vi "SLSC_Example_AsyscRTEnginer.vi"(10 "Parameters":variant, 11 "Process":refnum<class "Process.lvclass">) -> ()   [LabVIEW 2015, in "SLSC Module Template Engine.lvlib"]
uses:
  SLSC Module Template Engine.lvlib
  <vilib>/NI/NIVS Inline Async API/_VS Inline Async API/Process/Process.lvclass
  Shared/Compiled.Settings
  Shared/SLSC Dynamic Channel.ctl
  Types/Async Engine State Control.ctl
  <vilib>/NI/NIVS Inline Async API/_VS Inline Async API/Process/Process.lvclass/Process.ctl
  <vilib>/NI/NIVS Inline Async API/_Data Access Engine/Access Type Classes/Read/Read.lvclass/Read.ctl
  <vilib>/NI/NIVS Inline Async API/_Data Access Engine/Access Type Classes/ReadWrite/ReadWrite.lvclass/ReadWrite.ctl
  <vilib>/NI/NIVS Inline Async API/_Data Access Engine/Access Type Classes/Write/Write.lvclass/Write.ctl
  <vilib>/NI/NIVS Inline Async API/_Data Access Engine/Data Access Engine/Methods/Read.Data.vi
  <vilib>/NI/NIVS Inline Async API/_Data Access Engine/Data Access Engine/Methods/Write.Data.vi
  <vilib>/NI/NIVS Inline Async API/_Data Access Engine/Data Access Engine/Methods/ReadWrite.Data.vi
  <vilib>/NI/NIVS Inline Async API/_VS Inline Async API/Process/Data Member Access/Read Data Access.vi
  <vilib>/NI/NIVS Inline Async API/_VS Inline Async API/Error Handling Process/SubVIs/Error.ConvertArray.vi
  <vilib>/NI/NIVS Inline Async API/_Data Access Engine/Access Type Classes/Read/Read.ProcessData.vi
  <vilib>/NI/NIVS Inline Async API/_Data Access Engine/Access Type Classes/Write/Write.ProcessData.vi
  SLSC_Determine_Resource.vi
  <vilib>/NI/NIVS Inline Async API/_Data Access Engine/Access Type Classes/ReadWrite/ReadWrite.ProcessData.vi
  <vilib>/SLSC/Commit Properties.vi
  <vilib>/SLSC/Commit Properties for Devices.vi
  <vilib>/SLSC/Set Generic Property.vi
  <vilib>/SLSC/Set Generic Property (U64).vi
  <vilib>/SLSC/Set Generic Property (U32).vi
  <vilib>/SLSC/Set Generic Property (String).vi
  <vilib>/SLSC/Set Generic Property (I64).vi
  <vilib>/SLSC/Set Generic Property (I32).vi
  <vilib>/SLSC/Set Generic Property (DBL).vi
  <vilib>/SLSC/Set Generic Property (Bool).vi
  <vilib>/SLSC/Close Session.vi
  <vilib>/SLSC/Get Generic Property.vi
  <vilib>/SLSC/Get Generic Property (U64).vi
  <vilib>/SLSC/Get Generic Property (U32).vi
  <vilib>/SLSC/Get Generic Property (String).vi
  <vilib>/SLSC/Get Generic Property (I64).vi
  <vilib>/SLSC/Get Generic Property (I32).vi
  <vilib>/SLSC/Get Generic Property (DBL).vi
  <vilib>/SLSC/Get Generic Property (Bool).vi
  <vilib>/SLSC/Execute Command.vi
  <vilib>/SLSC/Execute Phys Chan Command.vi
  <vilib>/SLSC/Execute Device Command.vi
  <vilib>/NI/NIVS Inline Async API/_Data Access Engine/Data Access Engine/Methods/ReadWrite.Lookup.vi
  <vilib>/NI/NIVS Inline Async API/_Data Access Engine/Data Access Engine/Methods/Read.Lookup.vi
  <vilib>/NI/NIVS Inline Async API/_Data Access Engine/Data Access Engine/Methods/Write.Lookup.vi
  Shared/Constants.vi
  <vilib>/NI/NIVS Inline Async API/_Data Access Engine/Data Access Engine/Data Access Engine.lvclass
  <vilib>/NI Veristand/Custom Device Tools/Custom Device Utility Library/Custom Device Utility Library.lvlib
  <vilib>/SLSC/SLSC.lvlib
  Shared/SLSC Module Template Shared.lvlib
  System Explorer/SLSC Module Template System Explorer.lvlib
panel:
  in  "LoopRate(ms)":u32=50
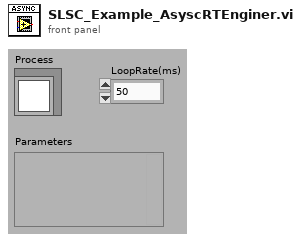
[diagram p1: front panel]
types:
  T1 = typedef "SLSC Module Template Engine.lvlib/Async Engine State Control.ctl" = enum16{"Initialize", "Configure", "Run", "Reset", "Shutdown"}
  T2 = typedef "SLSC Module Template Shared.lvlib/Compiled.Settings" = cluster{"Name":string, "SLSC IP Address":string, "Slot #":i32, "Configuration Data":cluster{"Properties":cluster{"Boolean Properties":cluster{"property":refnum<k21>, "Value":bool, "SLSC Item":refnum<k21>}[], "Double Properties":cluster{"property":refnum<k21>, "Double Write":dbl, "SLSC Item":refnum<k21>}[], "I32 Properties":cluster{"property":refnum<k21>, "Int32 Write":i32, "SLSC Item":refnum<k21>}[], "I64 Properties":cluster{"property":refnum<k21>, "Int64 Write":i64, "SLSC Item":refnum<k21>}[], "String Properties":cluster{"property":refnum<k21>, "String Write":string, "SLSC Item":refnum<k21>}[], "U32 Properties":cluster{"property":refnum<k21>, "UInt32 Write":u32, "SLSC Item":refnum<k21>}[], "U64 Properties":cluster{"property":refnum<k21>, "UInt64 Write":u64, "SLSC Item":refnum<k21>}[]}}, "SLSC Dynamic Inputs":T3[], "SLSC Dynamic Outputs":T3[], "SLSC Dynamic Commands":T3[]}
  T3 = typedef "SLSC Module Template System Explorer.lvlib/SLSC Dynamic Channel.ctl" = cluster{"SLSC Item":string, "property":string, "Data Type":enum16{"Bool", "Double", "I32", "I64", "String", "U32", "U64"}}
  T4 = typedef "Data Access Engine.lvlib/Data Access Engine.lvclass/Write.DVR.ctl" = refnum<data-value>
  T5 = typedef "Data Access Engine.lvlib/Data Access Engine.lvclass/Read.DVR.ctl" = refnum<data-value>
  T6 = typedef "Data Access Engine.lvlib/Data Access Engine.lvclass/ReadWrite.DVR.ctl" = refnum<data-value>
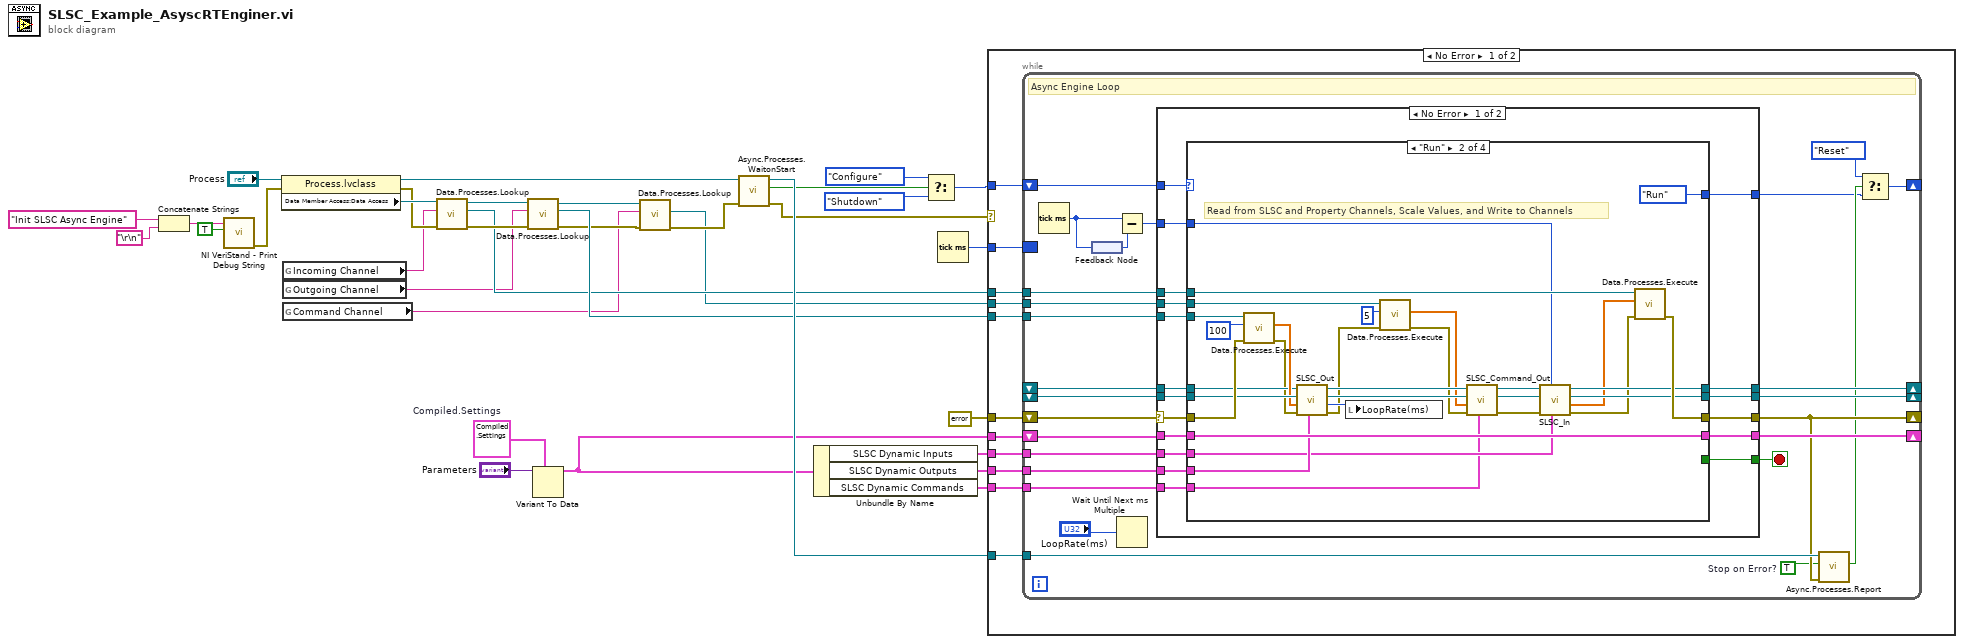
[diagram p0: block diagram]
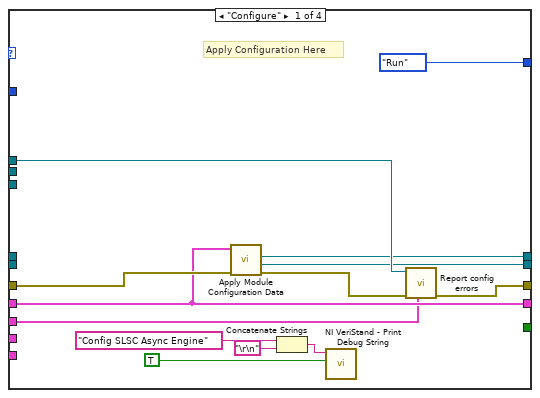
[diagram p2: hidden frame]
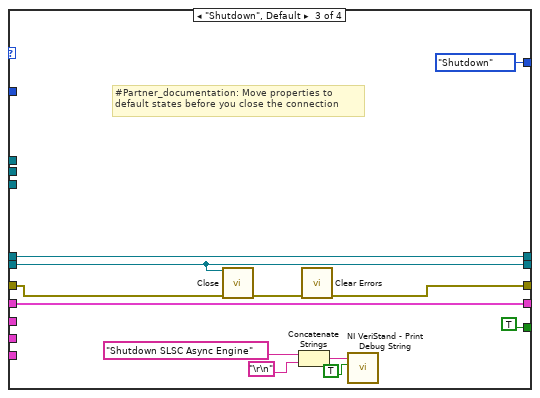
[diagram p3: hidden frame]
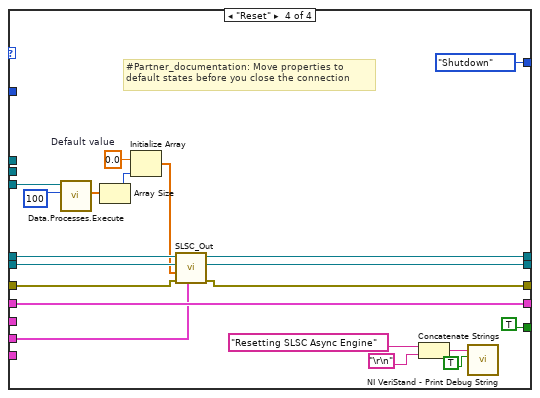
[diagram p4: hidden frame]
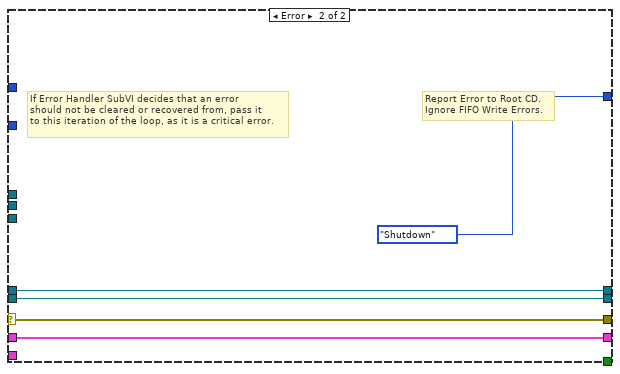
[diagram p5: hidden frame]
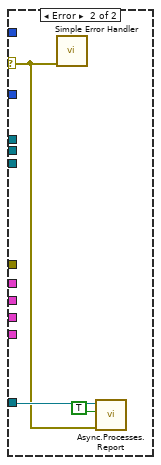
[diagram p6: hidden frame]
diagram:
  w23 = T2 {"Name"="", "SLSC IP Address"="", "Slot #"=0, "Configuration Data"={"Properties"={"Boolean Properties"=[], "Double Properties"=[], "I32 Properties"=[], "I64 Properties"=[], "String Properties"=[], "U32 Properties"=[], "U64 Properties"=[]}}, "SLSC Dynamic Inputs"=[], "SLSC Dynamic Outputs"=[], "SLSC Dynamic Commands"=[]}  # Compiled.Settings
  n1 = Concatenate Strings("Init SLSC Async Engine" ("Message"), "\r\n") -> (w20:string)
  n2 = call <vilib>:"NI VeriStand - Print Debug String.vi"("Add to log file? (T)"=TRUE, "Message"=w20) -> ("error out"=w7:errorcluster)  [unwired: 9 in]
  n3 = property class="Process.lvclass"(reference="Process", error in=w7) -> (reference out=w27:refnum<class "Process.lvclass">, error out=w25:errorcluster, "Data Member Access:Data Access"=w26:refnum<class "Data Access Engine.lvclass">)
  n4 = global read "Constants.vi" "Incoming Channel"() -> (w10:string)
  n5 = global read "Constants.vi" "Outgoing Channel"() -> (w9:string)
  n6 = global read "Constants.vi" "Command Channel"() -> (w2:string)
  n7 = call-poly <vilib>:"Data.Processes.Lookup.vi"("error in (no error)"=w25, "Name"=w10, "Data Access API in"=w26) -> ("error out"=w31:errorcluster, "Ref"=w30:T4, "Data Access API out"=w29:refnum<class "Data Access Engine.lvclass">)  [unwired: 5 in, 1 out]
  n8 = call-poly <vilib>:"Data.Processes.Lookup.vi"("error in (no error)"=w31, "Name"=w9, "Data Access API in"=w29) -> ("error out"=w4:errorcluster, "Ref"=w32:T5, "Data Access API out"=w5:refnum<class "Data Access Engine.lvclass">)  [unwired: 5 in, 1 out]
  n9 = Variant To Data(type=w23, Variant="Parameters") -> (data=w13:T2)  [unwired: 1 in, 1 out]
  n10 = call-poly <vilib>:"Data.Processes.Lookup.vi"("error in (no error)"=w4, "Name"=w2, "Data Access API in"=w5) -> ("error out"=w3:errorcluster, "Ref"=w1:T6)  [unwired: 5 in, 2 out]
  n11 = call <vilib>:"Async.Processes.WaitonStart.vi"("error in (no error)"=w3, "Process"=w27) -> ("error out"=w33:errorcluster, "Execute"=w17:bool, "Process out"=w34:refnum<class "Process.lvclass">)  [unwired: 7 in]
  n12 = Unbundle By Name(w13) -> ("SLSC Dynamic Inputs"=w12:T3[], "SLSC Dynamic Outputs"=w11:T3[], "SLSC Dynamic Commands"=w6:T3[])
  n13 = Select(t=Async_Engine_State_Control."Configure", s=w17, f=Async_Engine_State_Control."Shutdown") -> (s? t:f=w14:T1)
  n14 = Tick Count (ms)() -> (millisecond timer value=w8:u32)
  n15 = case shown="No Error" w33 {
    selector: w33 -> [_ w171]
    tunnel: w34 -> [w45 w172]
    tunnel: w30 -> [w44 _]
    tunnel: w32 -> [w43 _]
    tunnel: w13 -> [w37 _]
    tunnel: errorcluster {"status"=FALSE, "code"=0, "source"=""} ("error IO") -> [w42 _]
    tunnel: w14 -> [w41 _]
    tunnel: w12 -> [w40 _]
    tunnel: w11 -> [w39 _]
    tunnel: w8 -> [w38 _]
    tunnel: w6 -> [w36 _]
    tunnel: w1 -> [w35 _]
    frame No Error {
      n16 = while {
        shift-right: [w61] -> _
        shift-left: w42 -> [w70]
        shift-right: [w49] -> _
        shift-left: w41 -> [w69]
        shift-right: [w68] -> _
        shift-left: w37 -> [w67]
        shift-right: [w66] -> _
        shift-left: _ -> [w65]
        tunnel: w43 -> [w64]
        tunnel: w44 -> [w63]
        tunnel: w45 -> [w62]
        tunnel: w40 -> [w60]
        tunnel: w39 -> [w59]
        shift-right: [w58] -> _
        shift-left: _ -> [w57]
        border: w38 -> [_]
        tunnel: w36 -> [w47]
        tunnel: w35 -> [w46]
        stop <- w52 stop-if-true
        w56 = TRUE  # Stop on Error?
        # "Async Engine Loop"
        n17 = Tick Count (ms)() -> (millisecond timer value=w55:u32)
        n18 = feedback-in #1(w55) -> ()
        n19 = feedback #1() -> (w54:u32)
        n20 = Subtract(x=w55, y=w54) -> (x-y=w53:u32)
        n21 = Wait Until Next ms Multiple(millisecond multiple="LoopRate(ms)") -> ()  [unwired: 1 out]
        n22 = case shown="No Error" w70 {
          selector: w70 -> [w88 w166]
          tunnel: [w81 w166] -> w61
          tunnel: w69 -> [w89 _]
          tunnel: [w82 Async_Engine_State_Control."Shutdown"] -> w50
          tunnel: [w87 _] -> w52
          tunnel: [w86 w169] -> w68
          tunnel: w67 -> [w85 w169]
          tunnel: [w84 w168] -> w66
          tunnel: w65 -> [w83 w168]
          tunnel: w64 -> [w80 _]
          tunnel: w63 -> [w79 _]
          tunnel: w60 -> [w78 _]
          tunnel: w59 -> [w77 _]
          tunnel: [w76 w165] -> w58
          tunnel: w57 -> [w75 w165]
          tunnel: w53 -> [w74 _]
          tunnel: w47 -> [w73 _]
          tunnel: w46 -> [w72 _]
          frame No Error {
            n23 = case shown="\"Run\"" w89 {
              tunnel: w88 -> [w102 w129 w133 w145]
              tunnel: [w93 w128 w136 w157] -> w81
              tunnel: [Async_Engine_State_Control."Run" Async_Engine_State_Control."Run" Async_Engine_State_Control."Shutdown" Async_Engine_State_Control."Shutdown"] -> w82
              tunnel: [_ _ TRUE TRUE] -> w87
              tunnel: [w96 w132 w143 w163] -> w86
              tunnel: w85 -> [w96 w132 w143 w163]
              tunnel: [w90 w120 w134 w150] -> w84
              tunnel: w83 -> [_ w125 w134 w151]
              tunnel: w80 -> [_ w130 _ w155]
              tunnel: w79 -> [w94 w126 _ _]
              tunnel: w78 -> [w92 w118 _ _]
              tunnel: w77 -> [_ w123 _ w154]
              tunnel: [w91 w121 w135 w152] -> w76
              tunnel: w75 -> [_ w122 w135 w153]
              tunnel: w74 -> [_ w116 _ _]
              tunnel: w73 -> [_ w106 _ _]
              tunnel: w72 -> [_ w114 _ _]
              frame "Configure" {
                # "Apply Configuration Here"
                n24 = call "Apply Module Configuration Data.vi"("Error In"=w102, "Compiled.Settings"=w96) -> ("Error Out"=w95:errorcluster, "Module Session Out"=w90:refnum<k21>, "SLSC Module Name"=w91:refnum<k21>)  [unwired: 6 in, 1 out]
                n25 = Concatenate Strings("Config SLSC Async Engine" ("Message"), "\r\n") -> (w98:string)
                n26 = call <vilib>:"NI VeriStand - Print Debug String.vi"("Add to log file? (T)"=TRUE, "Message"=w98) -> ()  [unwired: 9 in, 1 out]
                n27 = call "Report config errors.vi"("SLSC Dynamic Inputs"=w92, "error in (no error)"=w95, "Data Value Reference in"=w94) -> ("error out"=w93:errorcluster)  [unwired: 8 in]
              }
              frame "Run" {
                # "Read from SLSC and Property Channels, Scale Values, and Write to Channels"
                n28 = call-poly <vilib>:"Data.Processes.Execute.vi"("error in (no error)"=w129, "timeout ms"=100, "Ref"=w130) -> ("error out"=w105:errorcluster, "Values"=w124:dbl[])  [unwired: 6 in, 1 out]
                n29 = call "SLSC_Out.vi"("SLSC Dynamic Outputs"=w123, "error in"=w105, "Values"=w124, "session in"=w125, "SLSC Module Name"=w122) -> ("error out"=w104:errorcluster, "LoopRate(ms)"=w117:u32, "session out"=w111:refnum<k21>, "SLSC Module Name"=w112:refnum<k21>)  [unwired: 3 in]
                n30 = local write "LoopRate(ms)"(w117) -> ()
                n31 = call-poly <vilib>:"Data.Processes.Execute.vi"("error in (no error)"=w104, "timeout ms"=5, "Ref"=w114) -> ("error out"=w103:errorcluster, "Data"=w108:dbl[])  [unwired: 5 in, 2 out]
                n32 = call "SLSC_Command_Out.vi"("SLSC Dynamic Commands"=w106, "error in"=w103, "Values"=w108, "session in"=w111, "SLSC Module Name"=w112) -> ("error out"=w107:errorcluster, "session out"=w109:refnum<k21>, "SLSC Module Name"=w110:refnum<k21>)  [unwired: 4 in]
                n33 = call "SLSC_In.vi"("SLSC Dynamic Inputs"=w118, "LoopDuration(ms)"=w116, "error in"=w107, "session in"=w109, "SLSC Module Name"=w110) -> ("error out"=w119:errorcluster, "Values"=w115:dbl[], "session out"=w120:refnum<k21>, "SLSC Module Name"=w121:refnum<k21>)  [unwired: 3 in]
                n34 = call-poly <vilib>:"Data.Processes.Execute.vi"("error in (no error)"=w119, "Values"=w115, "Ref"=w126) -> ("error out"=w128:errorcluster)  [unwired: 8 in]
              }
              frame "Shutdown", Default {
                # "#Partner_documentation: Move properties to \ndefault states before you close the connection"
                n35 = call-poly <vilib>:"Close.vi"("session in"=w134, "error in (no error)"=w133) -> ("error out"=w137:errorcluster)  [unwired: 13 in]
                n36 = Concatenate Strings("Shutdown SLSC Async Engine" ("Message"), "\r\n") -> (w139:string)
                n37 = call <vilib>:"Clear Errors.vi"("error in (no error)"=w137) -> ("error out"=w136:errorcluster)  [unwired: 5 in, 1 out]
                n38 = call <vilib>:"NI VeriStand - Print Debug String.vi"("Add to log file? (T)"=TRUE, "Message"=w139) -> ()  [unwired: 9 in, 1 out]
              }
              frame "Reset" {
                w147 = 0.0  # Default value
                # "#Partner_documentation: Move properties to \ndefault states before you close the connection"
                n39 = call-poly <vilib>:"Data.Processes.Execute.vi"("timeout ms"=100, "Ref"=w155) -> ("Values"=w149:dbl[])  [unwired: 7 in, 2 out]
                n40 = Array Size(array=w149) -> (size(s)=w148:i32)
                n41 = Initialize Array(w147, w148) -> (w146:dbl[])
                n42 = call "SLSC_Out.vi"("SLSC Dynamic Outputs"=w154, "error in"=w145, "Values"=w146, "session in"=w151, "SLSC Module Name"=w153) -> ("error out"=w157:errorcluster, "session out"=w150:refnum<k21>, "SLSC Module Name"=w152:refnum<k21>)  [unwired: 3 in, 1 out]
                n43 = Concatenate Strings("Resetting SLSC Async Engine" ("Message"), "\r\n") -> (w159:string)
                n44 = call <vilib>:"NI VeriStand - Print Debug String.vi"("Add to log file? (T)"=TRUE, "Message"=w159) -> ()  [unwired: 9 in, 1 out]
              }
            }
          }
          frame Error {
            # "If Error Handler SubVI decides that an error\nshould not be cleared or recovered from, pass it\nto this iteration of the loop, as it is a critical error."
            # "Report Error to Root CD.\nIgnore FIFO Write Errors."
          }
        }
        n45 = call <vilib>:"Async.Processes.Report.vi"("Error"=w61, "Stop Async on Error?"=w56, "Process in"=w62) -> ("Stop"=w51:bool)  [unwired: 7 in, 1 out]
        n46 = Select(t=Async_Engine_State_Control."Reset", s=w51, f=w50) -> (s? t:f=w49:T1)
      }
    }
    frame Error {
      n47 = call <vilib>:"Simple Error Handler.vi"("error in (no error)"=w171) -> ()  [unwired: 4 in, 5 out]
      n48 = call <vilib>:"Async.Processes.Report.vi"("Error"=w171, "Stop Async on Error?"=TRUE ("Stop on Error?"), "Process in"=w172) -> ()  [unwired: 7 in, 2 out]
    }
  }
